vi "save channels to stacked tiff series.vi"(8 "frame number in":i32, 9 "last frame":bool, 11 "image data in":dbl[][](array[numeric])) -> ()   [LabVIEW 2012]
doc: "SciScan 1.2 160622"
uses:
  Custom Controls/file format type def.ctl
  GFG/GFGpathGet.vi
  GFG/GFGnumericGet.vi
  GFG/GFGstringGet.vi
  Libtiff3/libtiff3.llb/libtiff3.lvlib
  GFG/GFG library.lvlib
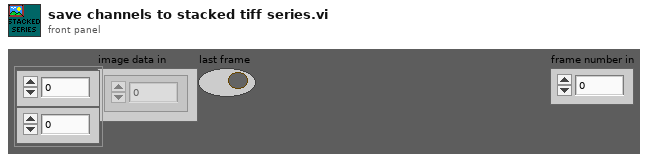
[diagram p1: front panel]
types:
  T1 = typedef "file format type def.ctl" = enum16{"16bit raw", "32bit raw", "16bit multi-tiff (interleave)", "16bit multi-tiff (separate)", "16bit multi-tiff (stacked)", "32bit multi-tiff (interleave)", "32bit multi-tiff (separate)", "32bit multi-tiff (stacked)", "16bit tiff series (interleave)", "16bit tiff series (separate)", "16bit tiff series (stacked)", "32bit tiff series (interleave)", "32bit tiff series (separate)", "32bit tiff series (stacked)"}
  T2 = cluster{"no..of.frames.to.acquire":dbl, "x.pixels":dbl, "y.pixels":dbl, "x.pixel.sz":dbl, "y.pixel.sz":dbl}
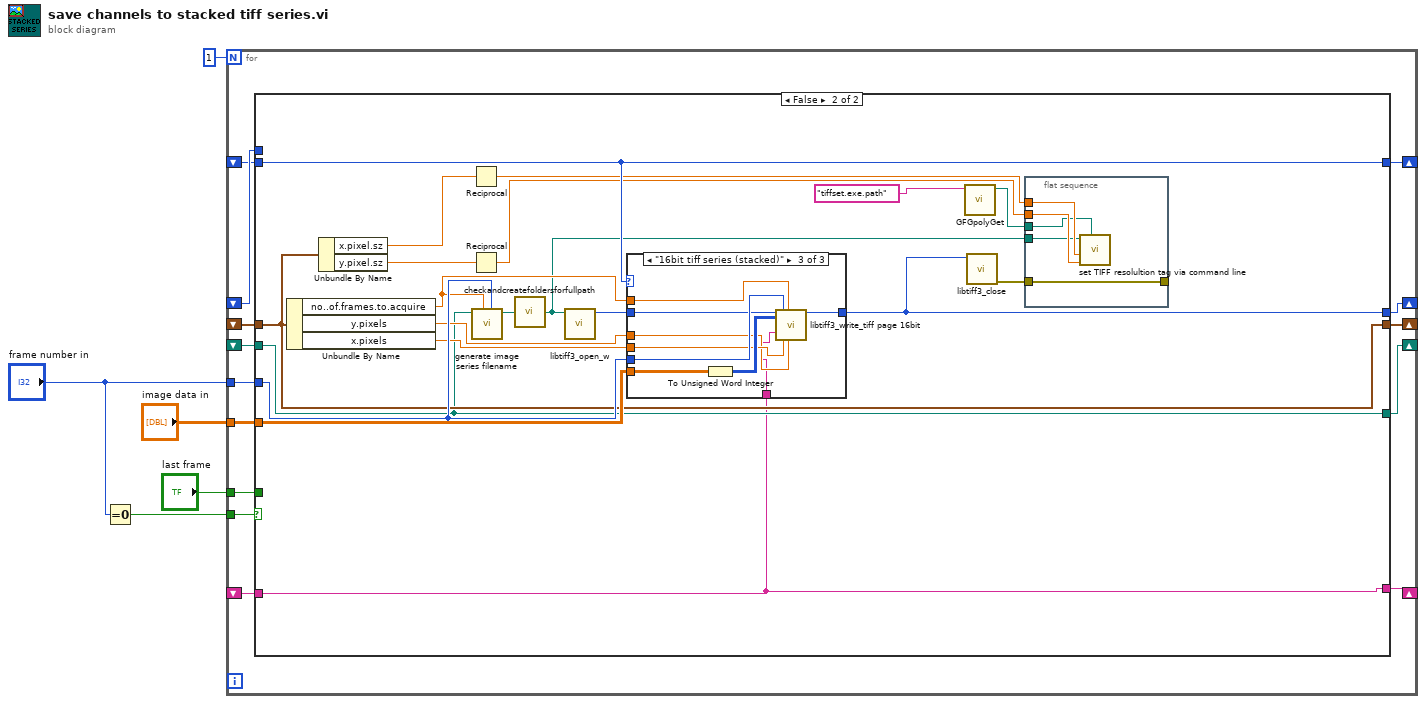
[diagram p0: block diagram]
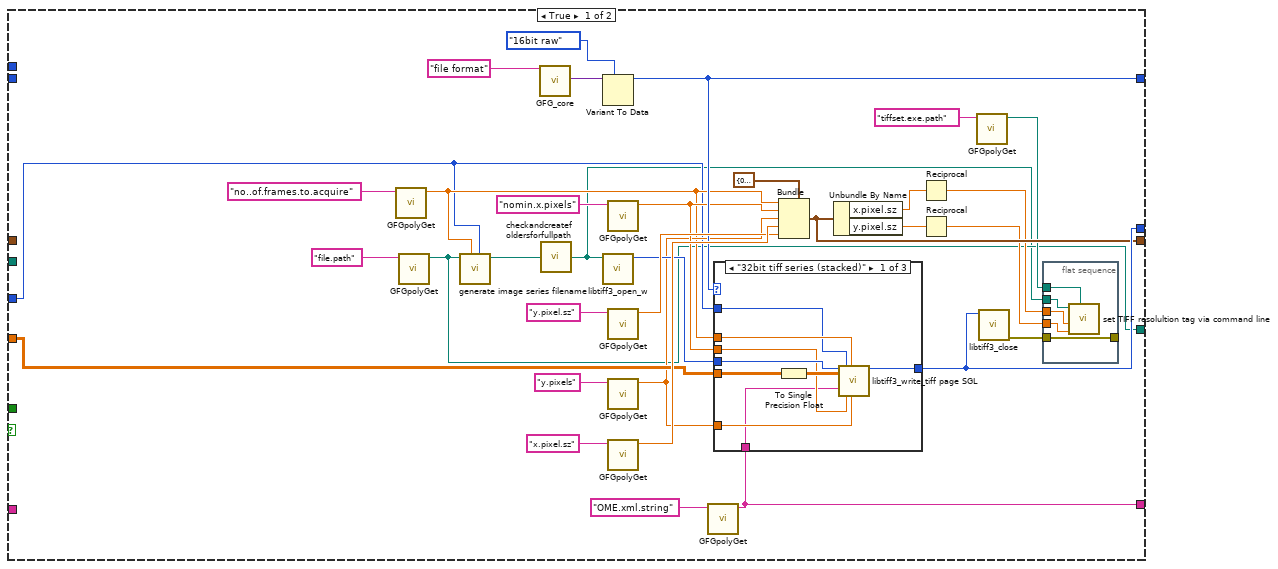
[diagram p2: hidden frame]
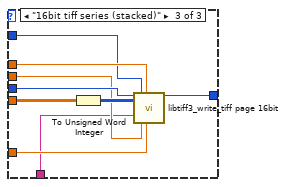
[diagram p4: hidden frame]
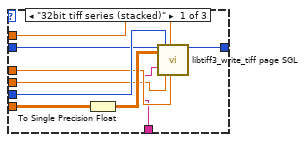
[diagram p5: hidden frame]
diagram:
  n1 = Equal To 0?(x="frame number in") -> (x = 0?=w4:bool)
  n2 = for {
    N: 1 -> [_]
    tunnel: w4 -> [w19]
    shift-right: [w18] -> _
    shift-left: _ -> [w17]
    tunnel: "image data in" -> [w16]
    shift-right: [w15] -> _
    shift-left: _ -> [w14]
    shift-right: [w13] -> _
    shift-left: _ -> [w12]
    shift-right: [w11] -> _
    shift-left: _ -> [w10]
    tunnel: "last frame" -> [w9]
    tunnel: "frame number in" -> [w8]
    shift-right: [w7] -> _
    shift-left: _ -> [w6]
    n3 = case shown="False" w19 {
      tunnel: w14 -> [_ w91]
      tunnel: [w32 w87] -> w18
      tunnel: w17 -> [_ _]
      tunnel: w16 -> [w39 w93]
      tunnel: [w40 w91] -> w15
      tunnel: [w31 w88] -> w13
      tunnel: w12 -> [_ w88]
      tunnel: [w23 w79] -> w11
      tunnel: w10 -> [_ w79]
      tunnel: w9 -> [_ _]
      tunnel: w8 -> [w33 w94]
      tunnel: [w20 w77] -> w7
      tunnel: w6 -> [_ w77]
      frame True {
        n4 = call-poly "GFGpolyGet.vi"("Variable Name in"="no..of.frames.to.acquire") -> ("Numeric"=w34:dbl)  [unwired: 8 in, 2 out]
        n5 = call-poly "GFGpolyGet.vi"("Variable Name in"="file.path") -> ("Path"=w23:path)  [unwired: 8 in, 2 out]
        n6 = call "generate image series filename.vi"("frame number in"=w33, "no..of.frames.to.acquire"=w34, "Path IN"=w23) -> ("appended path"=w35:path)  [unwired: 8 in]
        n7 = call "GFG_core.vi"("Variable Name in"="file format") -> ("Variant Out"=w51:variant)  [unwired: 12 in, 6 out]
        n8 = call "checkandcreatefoldersforfullpath.vi"("Path IN"=w35) -> ("Path OUT"=w22:path)  [unwired: 4 in]
        n9 = Variant To Data(type=file_format_type_def."16bit raw" ("file format"), Variant=w51) -> (data=w40:T1)  [unwired: 1 in, 1 out]
        n10 = call "libtiff3_open_w.vi"("Input path"=w22) -> ("handle"=w38:i32)  [unwired: 9 in, 1 out]
        n11 = call-poly "GFGpolyGet.vi"("Variable Name in"="nomin.x.pixels" ("Tag in")) -> ("Numeric"=w37:dbl)  [unwired: 8 in, 2 out]
        n12 = call-poly "GFGpolyGet.vi"("Variable Name in"="y.pixel.sz" ("Tag in")) -> ("Numeric"=w42:dbl)  [unwired: 8 in, 2 out]
        n13 = call-poly "GFGpolyGet.vi"("Variable Name in"="y.pixels" ("Tag in")) -> ("Numeric"=w36:dbl)  [unwired: 8 in, 2 out]
        n14 = call-poly "GFGpolyGet.vi"("Variable Name in"="x.pixel.sz" ("Tag in")) -> ("Numeric"=w43:dbl)  [unwired: 8 in, 2 out]
        n15 = call-poly "GFGpolyGet.vi"("Variable Name in"="OME.xml.string" ("Tag in")) -> ("String"=w20:string)  [unwired: 9 in, 1 out]
        n16 = case shown="\"32bit tiff series (stacked)\"" w40 {
          tunnel: w39 -> [w62 _ w73]
          tunnel: w38 -> [w63 w67 w74]
          tunnel: w33 -> [w64 _ w75]
          tunnel: w34 -> [w65 _ w76]
          tunnel: [w66 w67 w69] -> w32
          tunnel: w37 -> [w59 _ w71]
          tunnel: w36 -> [w60 _ w70]
          tunnel: w20 -> [w58 _ w68]
          frame "32bit tiff series (stacked)" {
            n17 = To Single Precision Float(number=w62) -> (single precision float=w61:sgl[][])
            n18 = call "libtiff3_write_tiff page SGL.vi"("Handle"=w63, "Image Pixels (Float)"=w61, "Image Description"=w58, "page"=w64, "x.pixels"=w59, "totalpages"=w65, "y.pixels"=w60) -> ("Handle out"=w66:i32)  [unwired: 11 in, 1 out]
          }
          frame Default {
          }
          frame "16bit tiff series (stacked)" {
            n19 = To Unsigned Word Integer(number=w73) -> (unsigned 16bit integer=w72:u16[][])
            n20 = call "libtiff3_write_tiff page 16bit.vi"("Handle"=w74, "Image Pixels (U16)"=w72, "ImageDescription"=w68, "page"=w75, "x.pixels"=w71, "totalpages"=w76, "y.pixels"=w70) -> ("Handle out"=w69:i32)  [unwired: 11 in, 1 out]
          }
        }
        n21 = Bundle(cluster=T2 {"no..of.frames.to.acquire"=0.0, "x.pixels"=0.0, "y.pixels"=0.0, "x.pixel.sz"=0.0, "y.pixel.sz"=0.0} ("output cluster"), "no..of.frames.to.acquire"=w34, "x.pixels"=w37, "y.pixels"=w36, "x.pixel.sz"=w43, "y.pixel.sz"=w42) -> (w31:T2)
        n22 = Unbundle By Name(w31) -> ("x.pixel.sz"=w26:dbl, "y.pixel.sz"=w27:dbl)
        n23 = Reciprocal(x=w26) -> (1/x=w28:dbl)
        n24 = Reciprocal(x=w27) -> (1/x=w29:dbl)
        n25 = call-poly "GFGpolyGet.vi"("Variable Name in"="tiffset.exe.path") -> ("Path"=w24:path)  [unwired: 8 in, 2 out]
        n26 = call "libtiff3_close.vi"("Handle"=w32) -> ("error out"=w30:errorcluster)  [unwired: 9 in]
        n27 = flat-sequence {
          tunnel: w30 -> [w55]
          tunnel: w28 -> [w57]
          tunnel: w29 -> [w56]
          tunnel: [w55] -> _
          tunnel: w24 -> [w54]
          tunnel: w22 -> [w53]
          frame #0 {
            n28 = call "set TIFF resolultion tag via command line.vi"("tiffset.exe file path"=w54, "y pixels per m"=w56, "x pixels per m"=w57, "TIFF file path"=w53) -> ()  [unwired: 8 in]
          }
        }
      }
      frame False {
        n29 = Unbundle By Name(w88) -> ("no..of.frames.to.acquire"=w92:dbl, "y.pixels"=w90:dbl, "x.pixels"=w89:dbl)
        n30 = Unbundle By Name(w88) -> ("x.pixel.sz"=w82:dbl, "y.pixel.sz"=w83:dbl)
        n31 = Reciprocal(x=w82) -> (1/x=w84:dbl)
        n32 = Reciprocal(x=w83) -> (1/x=w85:dbl)
        n33 = call "generate image series filename.vi"("frame number in"=w94, "no..of.frames.to.acquire"=w92, "Path IN"=w79) -> ("appended path"=w95:path)  [unwired: 8 in]
        n34 = call "checkandcreatefoldersforfullpath.vi"("Path IN"=w95) -> ("Path OUT"=w78:path)  [unwired: 4 in]
        n35 = call "libtiff3_open_w.vi"("Input path"=w78) -> ("handle"=w96:i32)  [unwired: 9 in, 1 out]
        n36 = case shown="\"16bit tiff series (stacked)\"" w91 {
          tunnel: w93 -> [w106 _ w117]
          tunnel: w96 -> [w107 w111 w118]
          tunnel: w94 -> [w108 _ w119]
          tunnel: w92 -> [w109 _ w120]
          tunnel: [w110 w111 w113] -> w87
          tunnel: w89 -> [w103 _ w115]
          tunnel: w90 -> [w104 _ w114]
          tunnel: w77 -> [w102 _ w112]
          frame "32bit tiff series (stacked)" {
            n37 = To Single Precision Float(number=w106) -> (single precision float=w105:sgl[][])
            n38 = call "libtiff3_write_tiff page SGL.vi"("Handle"=w107, "Image Pixels (Float)"=w105, "Image Description"=w102, "page"=w108, "x.pixels"=w103, "totalpages"=w109, "y.pixels"=w104) -> ("Handle out"=w110:i32)  [unwired: 11 in, 1 out]
          }
          frame Default {
          }
          frame "16bit tiff series (stacked)" {
            n39 = To Unsigned Word Integer(number=w117) -> (unsigned 16bit integer=w116:u16[][])
            n40 = call "libtiff3_write_tiff page 16bit.vi"("Handle"=w118, "Image Pixels (U16)"=w116, "ImageDescription"=w112, "page"=w119, "x.pixels"=w115, "totalpages"=w120, "y.pixels"=w114) -> ("Handle out"=w113:i32)  [unwired: 11 in, 1 out]
          }
        }
        n41 = call-poly "GFGpolyGet.vi"("Variable Name in"="tiffset.exe.path") -> ("Path"=w80:path)  [unwired: 8 in, 2 out]
        n42 = call "libtiff3_close.vi"("Handle"=w87) -> ("error out"=w86:errorcluster)  [unwired: 9 in]
        n43 = flat-sequence {
          tunnel: w86 -> [w99]
          tunnel: w84 -> [w101]
          tunnel: w85 -> [w100]
          tunnel: [w99] -> _
          tunnel: w80 -> [w98]
          tunnel: w78 -> [w97]
          frame #0 {
            n44 = call "set TIFF resolultion tag via command line.vi"("tiffset.exe file path"=w98, "y pixels per m"=w100, "x pixels per m"=w101, "TIFF file path"=w97) -> ()  [unwired: 8 in]
          }
        }
      }
    }
  }
